vi "CreateReportFolder.vi"(8 "error in (no error)":errorcluster) -> (0 "error out":errorcluster, 2 "ConfigPath":path)   [LabVIEW 2018, in "GUI.lvclass"]
uses:
  GUI.lvclass
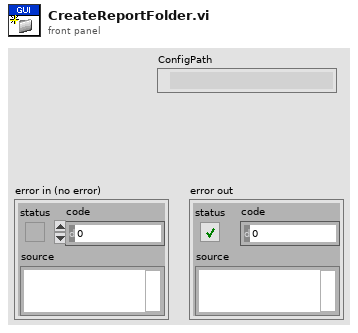
[diagram p1: front panel]
types:
  T1 = enum16{"open", "replace", "create", "open or create", "replace or create", "replace or create with confirmation"}
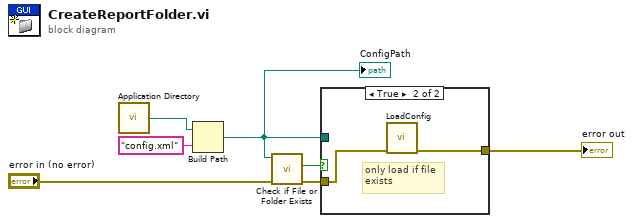
[diagram p0: block diagram]
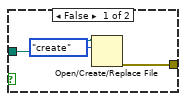
[diagram p2: hidden frame]
diagram:
  n1 = call <vilib>:"Application Directory.vi"() -> ("Application Directory"=w7:path)
  n2 = Build Path(base path=w7, name or relative path="config.xml") -> (appended path=w4:path)
  "ConfigPath" <- w4
  n3 = call <vilib>:"Check if File or Folder Exists.vi"("error in (no error)"="error in (no error)", "path"=w4) -> ("error out"=w1:errorcluster, "file or folder exists?"=w5:bool)  [unwired: 7 in, 1 out]
  n4 = case shown="True" w5 {
    tunnel: w4 -> [w10 _]
    tunnel: [w8 w12] -> w3
    tunnel: w1 -> [_ w11]
    frame False {
      n5 = Open/Create/Replace File(file path (use dialog)=w10, operation (0:open)=T1."create") -> (error out=w8:errorcluster)  [unwired: 4 in, 2 out]
    }
    frame True {
      # "only load if file\nexists"
      n6 = call "LoadConfig.vi"("error in"=w11) -> ("error out"=w12:errorcluster)  [unwired: 10 in]
    }
  }
  "error out" <- w3
